vi "analog trigger initial.vi"(7 "sample mode":i32(ring)=10178 caption="샘플 모드" items=["유한 샘플"=10178, "연속 샘플"=10123, "하드웨어 타이밍에 의한 단일 포인트"=12522], 8 "error in":errorcluster caption="에러 입력", 9 "samples per channel":i32=1000 caption="채널당 샘플", 10 "rate":dbl=1000.0 caption="속도" format="%0.2f", 11 "physical channels":tag caption="물리적 채널") -> (0 "error out":errorcluster caption="에러 출력", 3 "task out":refnum<k21> caption="태스크 출력")   [LabVIEW 2013]
uses:
  <vilib>/DAQmx/create/channels.llb/DAQmx Create Channel (DI-Digital Input).vi
  <vilib>/DAQmx/configure/timing.llb/DAQmx Timing (Sample Clock).vi
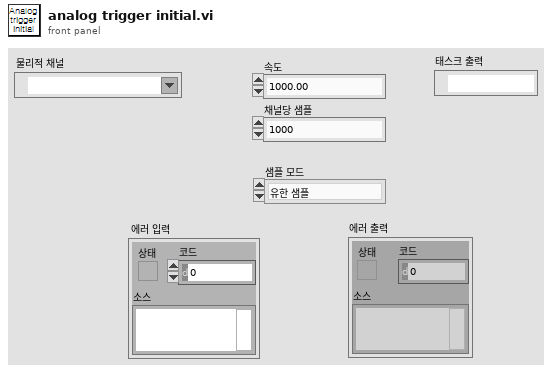
[diagram p1: front panel]
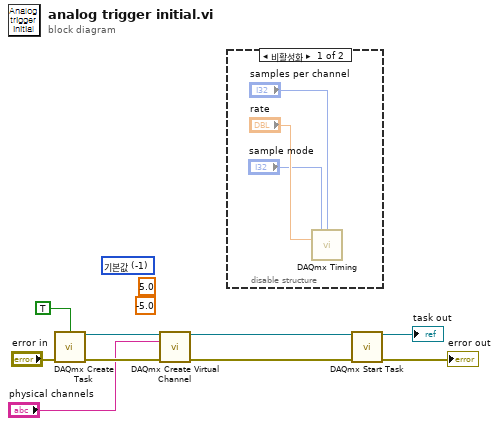
[diagram p0: block diagram]
diagram:
  (unwired) -1 items=["기본값"=-1, "RSE"=10083, "NRSE"=10078, "차동"=10106, "유사 차동"=12529] ("input terminal configuration")
  (unwired) 5.0 ("maximum value")
  (unwired) -5.0 ("minimum value")
  n1 = call <vilib>:"DAQmx Create Task.vi"("auto cleanup"=TRUE, "error in"="error in") -> ("task out"=w8:refnum<k21>, "error out"=w9:errorcluster)  [unwired: 12 in]
  n2 = call-poly <vilib>:"DAQmx Create Virtual Channel.vi"("task in"=w8, "lines"="physical channels", "error in"=w9) -> ("task out"=w2:refnum<k21>, "error out"=w1:errorcluster)  [unwired: 11 in]
  n3 = disable-structure shown="비활성화" {
    frame Disabled {
      n4 = call-poly <vilib>:"DAQmx Timing.vi"("sample mode"="sample mode", "samples per channel"="samples per channel", "rate"="rate") -> ()  [unwired: 11 in, 2 out]
    }
    frame Enabled {
    }
  }
  n5 = call <vilib>:"DAQmx Start Task.vi"("task/channels in"=w2, "error in"=w1) -> ("task out"=→"task out":refnum<k21>, "error out"=→"error out":errorcluster)  [unwired: 12 in]
